vi "read.vi"(8 "error in":errorcluster, 11 "Text Session in":refnum<class "Text Device Session.lvclass">) -> (0 "error out":errorcluster, 2 "Data Out":string, 3 "Text Session out":refnum<class "Text Device Session.lvclass">)   [LabVIEW 2015, in "Text Device Session.lvclass"]
uses:
  Text Device Session.lvclass
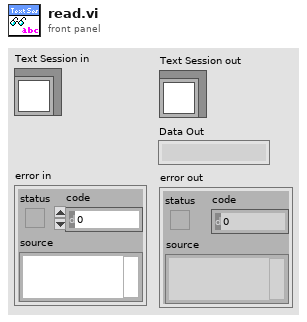
[diagram p1: front panel]
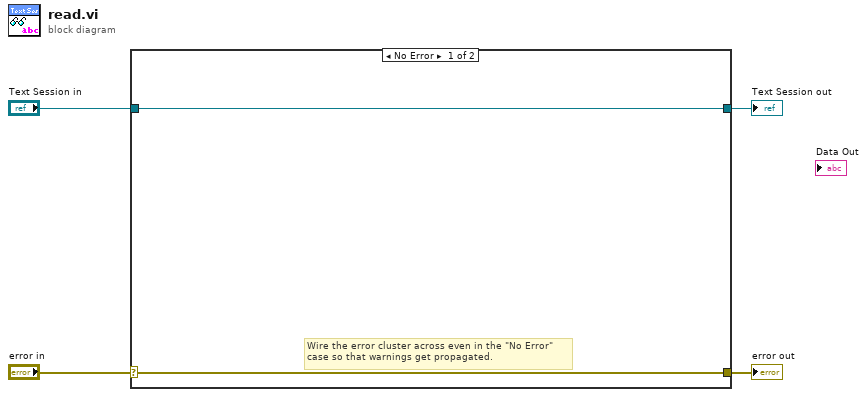
[diagram p0: block diagram]
diagram:
  n1 = case shown="No Error" "error in" {
    selector: "error in" -> [w5 w8]
    tunnel: [w5 w8] -> w3
    tunnel: [w6 w7] -> w1
    tunnel: "Text Session in" -> [w6 w7]
    frame No Error {
      # "Wire the error cluster across even in the \"No Error\"\ncase so that warnings get propagated."
    }
    frame Error {
    }
  }
  "error out" <- w3
  "Text Session out" <- w1
